vi "TextControlledInstrumControlToCommand.vi"   [LabVIEW 2019]
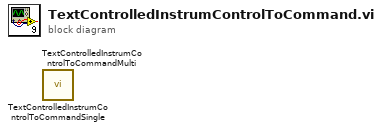
[diagram p0: block diagram]
diagram:
  n1 = call "TextControlledInstrumControlToCommandSingle.vi"() -> ()  [unwired: 11 in, 1 out]
  n2 = call "TextControlledInstrumControlToCommandMulti.vi"() -> ()  [unwired: 11 in, 1 out]
